vi "Untitled 1.vi"() -> ()   [LabVIEW 2021]
uses:
  <vilib>/measure/NI_MABase.lvlib
panel:
  in  "offset 2":dbl format="%0.2p"
  out "signal out":waveform(dbl)
  out "phase out":dbl format="%.2p"
  out "error out":errorcluster
  in  "frequency":dbl=10.0 format="%0.2p"
  in  "amplitude":dbl=1.0 format="%0.2p"
  in  "phase":dbl format="%.2p"
  in  "error in (no error)":errorcluster
  in  "signal type":T1(ring)
  in  "sampling info":cluster{"Fs":dbl, "#s":dbl}={"Fs"=1000.0, "#s"=1000.0} {"Fs" format="%.2p"}
  in  "reset signal":bool
  in  "square wave duty cycle (%)":dbl=50.0 format="%0.2f"
  in  "offset":dbl format="%0.2p"
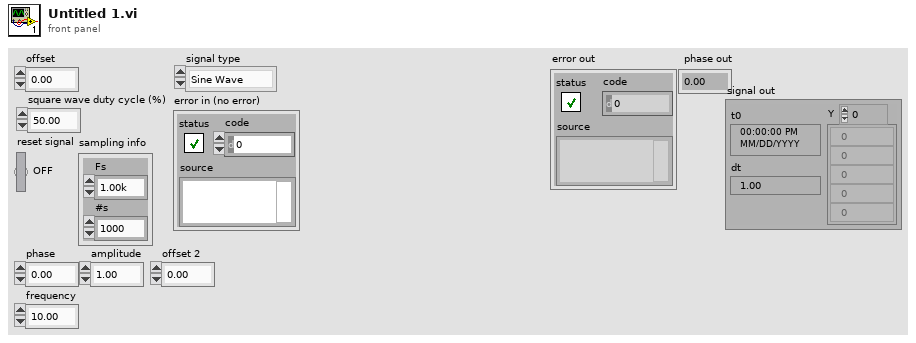
[diagram p1: front panel]
types:
  T1 = enum16{"Sine Wave", "Triangle Wave", "Square Wave", "Sawtooth Wave"}
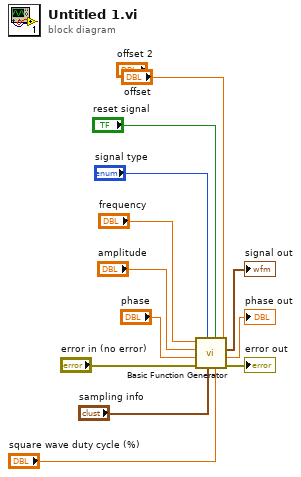
[diagram p0: block diagram]
diagram:
  n1 = call <vilib>:"Basic Function Generator.vi"("offset"="offset", "square wave duty cycle (%)"="square wave duty cycle (%)", "reset signal"="reset signal", "sampling info"="sampling info", "signal type"="signal type", "error in (no error)"="error in (no error)", "phase"="phase", "amplitude"="amplitude", "frequency"="frequency") -> ("error out"=→"error out":errorcluster, "phase out"=→"phase out":dbl, "signal out"=→"signal out":waveform(dbl))
